vi "TopMenu.vi"() -> ()   [LabVIEW 2011]
panel:
  out "strResultArrayOut":string[](array[string])
  in  "写指令":bool=TRUE
  in  "strModelChoice":string(combo)="WD5500"
  in  "VISA resource name":refnum<visa-resource-name>="COM1" caption="VISA资源名称"
  # "1号机"
  # "3号机"
  # "2号机"
  # "4号机"
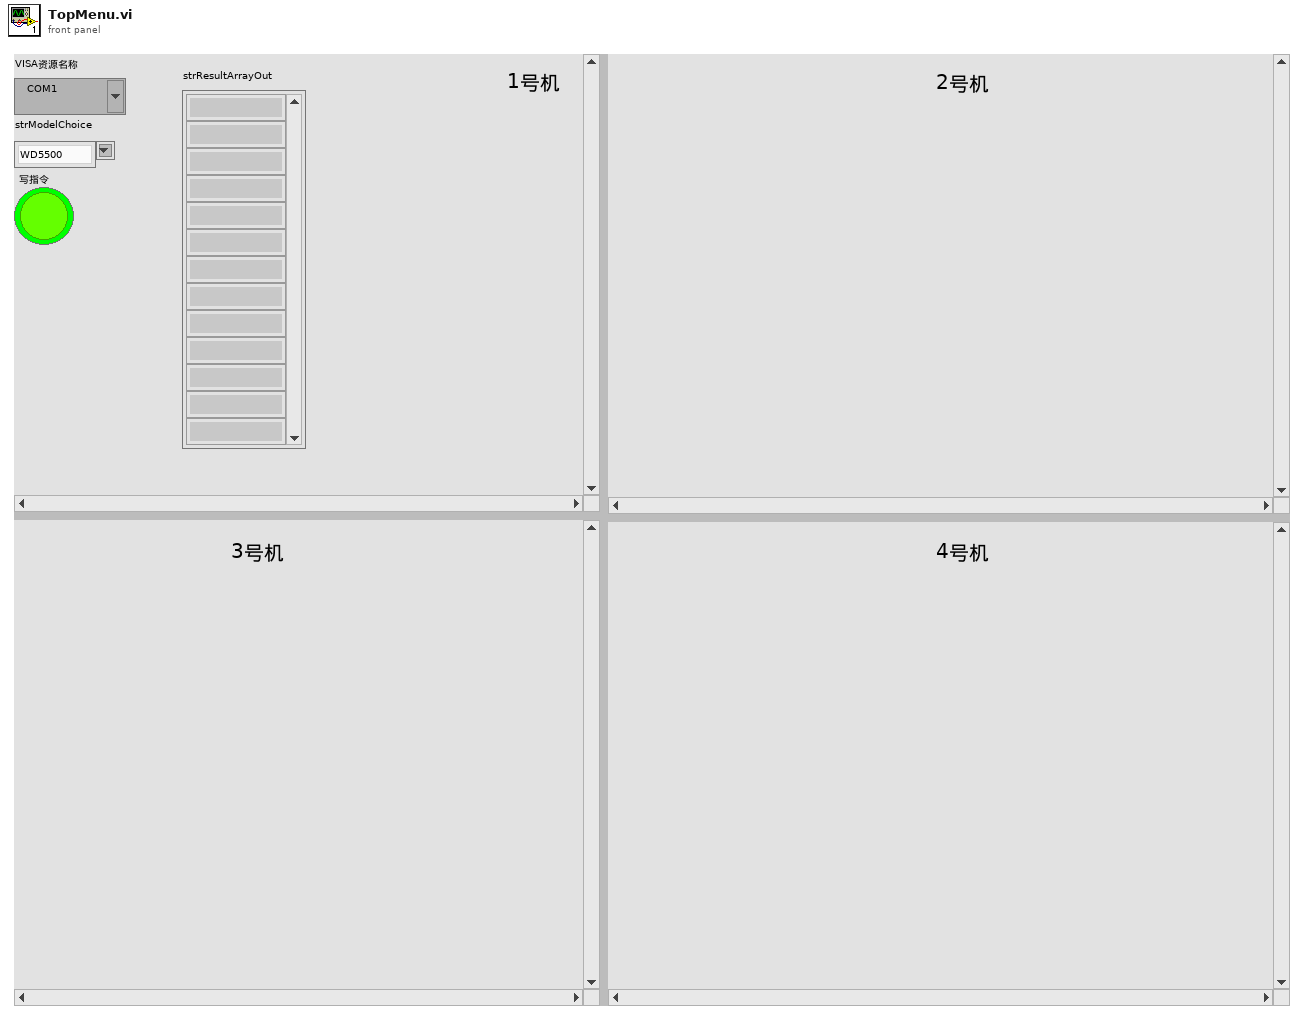
[diagram p1: front panel]
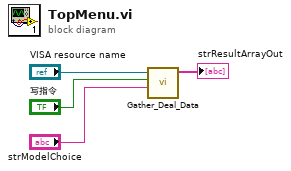
[diagram p0: block diagram]
diagram:
  n1 = call "Gather_Deal_Data.vi"("strModelChoice"="strModelChoice", "写指令"="写指令", "1号机端口"="VISA resource name") -> ("strResultArrayOut"=→"strResultArrayOut":string[])  [unwired: 6 in, 1 out]
